vi "Start Sync.vi"(8 "error in (no error)":errorcluster, 11 "gRPC Server in":refnum<class "TestServer.lvclass">) -> (0 "error out":errorcluster, 3 "gRPC Server out":refnum<class "TestServer.lvclass">)   [LabVIEW 2019, in "TestServer.lvlib" / "TestServer.lvclass"]
uses:
  TestServer.lvclass
  TestServer.lvclass/TestServer.ctl
  RPC Messages/niScope_ReadContinuouslyResult/niScope_ReadContinuouslyResult_Data.ctl
  gRPC lvSupport/gprc-lvsupport.lvlib
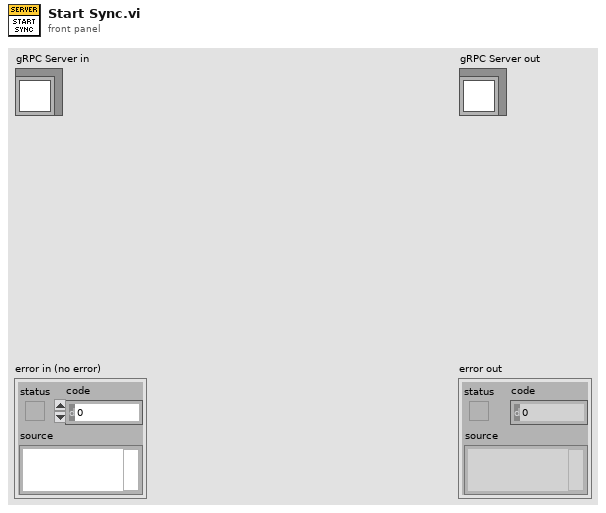
[diagram p1: front panel]
types:
  T1 = typedef "TestServer.lvlib/TestServer.lvclass/niScope_ReadContinuouslyResult_Data.ctl" = cluster{"status":i32, "wfm":dbl[]}
  T2 = typedef "TestServer.lvlib/TestServer.lvclass/Server gRPC UEs.ctl" = cluster{"StreamLatencyTest gRPC UE":refnum<user-event>, "StreamLatencyTestClient gRPC UE":refnum<user-event>, "StreamLatencyTestServer gRPC UE":refnum<user-event>, "Init gRPC UE":refnum<user-event>, "InitWithOptions gRPC UE":refnum<user-event>, "AutoSetup gRPC UE":refnum<user-event>, "ConfigureHorizontalTiming gRPC UE":refnum<user-event>, "TestWrite gRPC UE":refnum<user-event>, "Read gRPC UE":refnum<user-event>, "ReadContinuously gRPC UE":refnum<user-event>}
  T3 = typedef "TestServer.lvlib/gprc-lvsupport.lvlib/grpcId.ctl" = u64
  T4 = typedef "TestServer.lvlib/TestServer.lvclass/niScope_InitParameters_Data.ctl" = cluster{"id":i32}
  T5 = typedef "TestServer.lvlib/TestServer.lvclass/niScope_ReadContinuouslyParameters_Data.ctl" = cluster{"vi":T6, "channelList":string, "timeout":dbl, "numSamples":i32}
  T6 = typedef "TestServer.lvlib/TestServer.lvclass/niScope_ViSession_Data.ctl" = cluster{"id":u32}
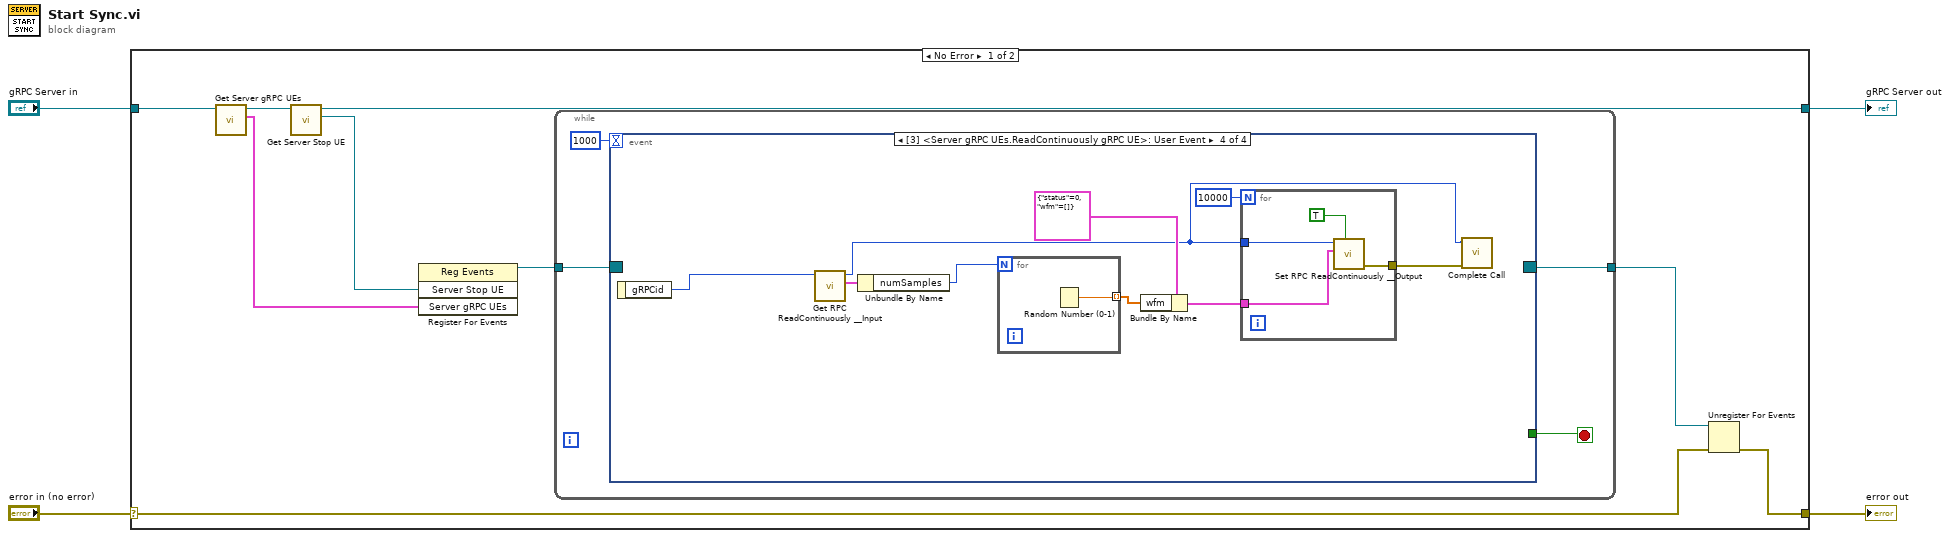
[diagram p0: block diagram]
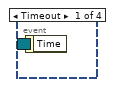
[diagram p2: hidden frame]
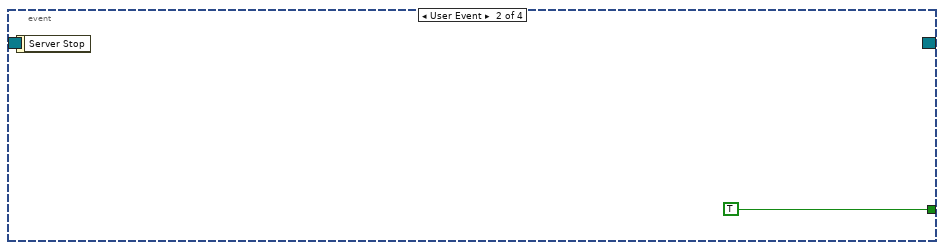
[diagram p3: hidden frame]
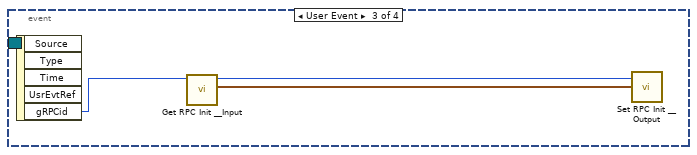
[diagram p4: hidden frame]
diagram:
  n1 = case shown="No Error" "error in (no error)" {
    selector: "error in (no error)" -> [w6 w37]
    tunnel: [w5 w37] -> w3
    tunnel: [w9 w36] -> w1
    tunnel: "gRPC Server in" -> [w13 w36]
    frame No Error {
      n2 = call "Get Server gRPC UEs.vi"("OOP Server in"=w13) -> ("Server gRPC UEs"=w10:T2, "OOP Server out"=w12:refnum<class "TestServer.lvclass">)  [unwired: 9 in]
      n3 = call "Get Server Stop UE.vi"("OOP Server in"=w12) -> ("Server Stop UE"=w11:refnum<user-event>, "OOP Server out"=w9:refnum<class "TestServer.lvclass">)  [unwired: 9 in]
      n4 = register-events(w11, w10) -> (reference out=w8:refnum<event-registration>)  [unwired: 2 in, 1 out]
      n5 = while {
        tunnel: w8 -> [w17]
        tunnel: [w15] -> w7
        stop <- w16 stop-if-true
        n6 = event "RPC Methods Event Structure" shown="[3] <Server gRPC UEs.ReadContinuously gRPC UE>: User Event" {
          selector: w17 -> [_ _ _ _]
          dyn-events: [_ _ _ _] -> w15
          timeout: 1000 -> [_ _ _ _]
          tunnel: [_ TRUE _ _] -> w16
          event Timeout {
            n7 = event-data() -> ()  [unwired: 1 in, 1 out]
          }
          event User Event {
            n8 = event-data() -> ()  [unwired: 1 in, 1 out]
          }
          event User Event {
            n9 = event-data() -> ("gRPCid"=w21:T3)  [unwired: 1 in, 4 out]
            n10 = call "Get RPC Init __Input.vi"("gRPCid in"=w21) -> ("Message Data"=w19:T4, "gRPCid out"=w20:T3)  [unwired: 8 in, 1 out]
            n11 = call "Set RPC Init __Output.vi"("Message Data"=w19, "gRPCid in"=w20) -> ()  [unwired: 9 in, 1 out]
          }
          event User Event {
            n12 = event-data() -> ("gRPCid"=w30:T3)  [unwired: 1 in]
            n13 = call "Get RPC ReadContinuously __Input.vi"("gRPCid in"=w30) -> ("Message Data"=w29:T5, "gRPCid out"=w23:T3)  [unwired: 8 in, 1 out]
            n14 = Unbundle By Name(w29) -> ("numSamples"=w28:i32)
            n15 = for {
              N: w28 -> [_]
              tunnel: [w35] -> w27 mode=indexing
              n16 = Random Number (0-1)() -> (number: 0 to 1=w35:dbl)
            }
            n17 = Bundle By Name(cluster=T1 {"status"=0, "wfm"=[]} ("Message Data"), "wfm"=w27) -> (w25:T1)
            n18 = for {
              N: 10000 -> [_]
              tunnel: w23 -> [w33]
              tunnel: w25 -> [w34]
              tunnel: [w32] -> w22
              n19 = call "Set RPC ReadContinuously __Output.vi"("Streeming? (F)"=TRUE, "Message Data"=w34, "gRPCid in"=w33) -> ("error out"=w32:errorcluster)  [unwired: 8 in]
            }
            n20 = call "Complete Call.vi"("gRPCid"=w23, "error in (no error)"=w22) -> ()  [unwired: 8 in, 1 out]
          }
        }
      }
      n21 = Unregister For Events(event registration refnum=w7, error in=w6) -> (error out=w5:errorcluster)
    }
    frame Error {
    }
  }
  "error out" <- w3
  "gRPC Server out" <- w1
